vi "请双击登录.vi"() -> ()   [LabVIEW 2012]
panel:
  out "主VI路径":path
  out "注册状态提示":string
  in  "注册":bool
  in  "登录":bool
  in  "退出":bool
  in  "密    码":string
  in  "用户名":string
  out "数值":i32
  out "路径":path=path "D:/labVIs/0921/用户数据.txt"
  # "说明：请先输入用户名和密码再点击注册或登录\n默认用户名：20154207         密码：20154207"
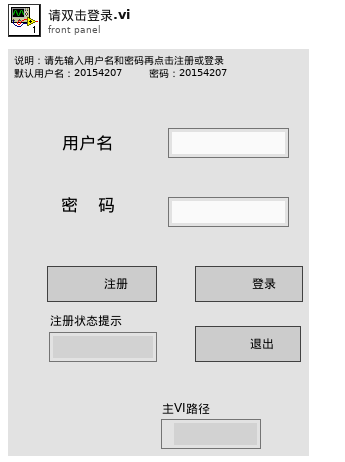
[diagram p1: front panel]
types:
  T1 = enum16{"open", "replace", "create", "open or create", "replace or create", "replace or create with confirmation"}
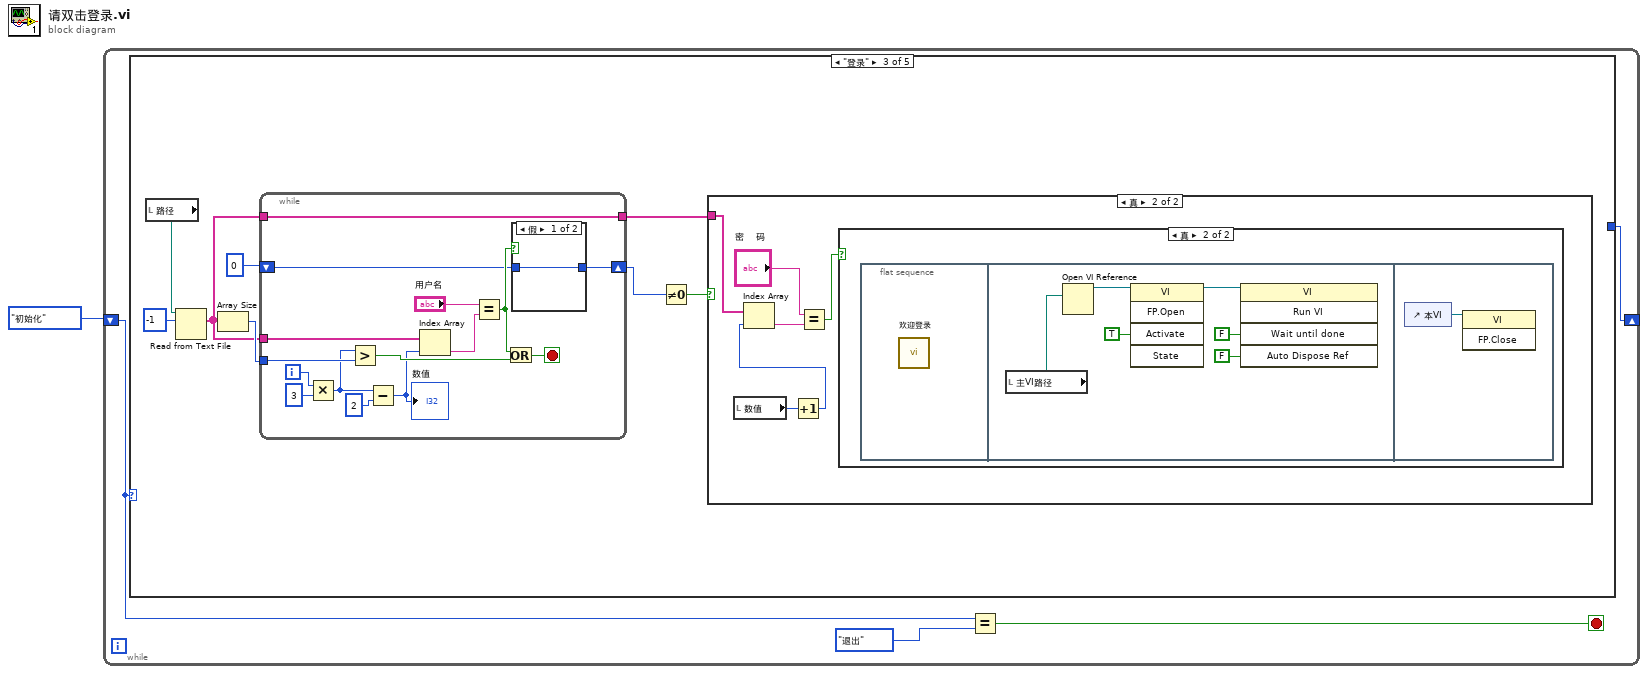
[diagram p0: block diagram]
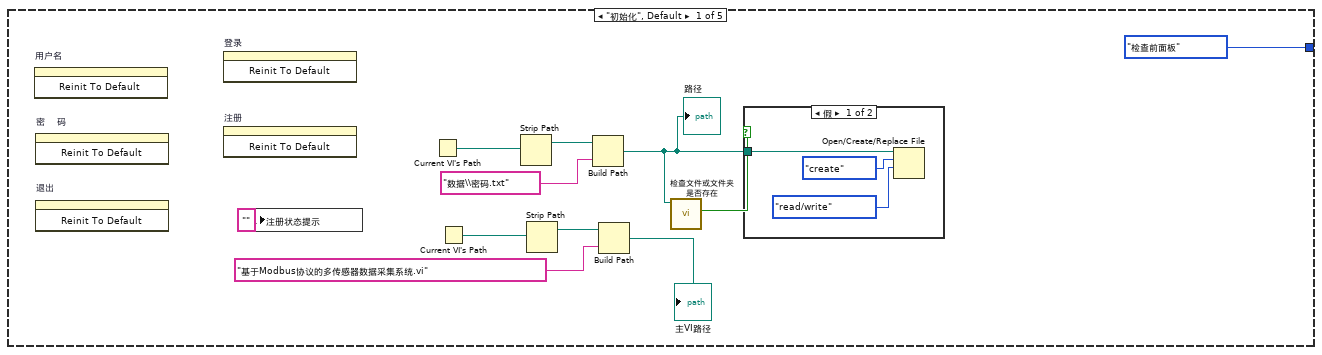
[diagram p2: hidden frame]
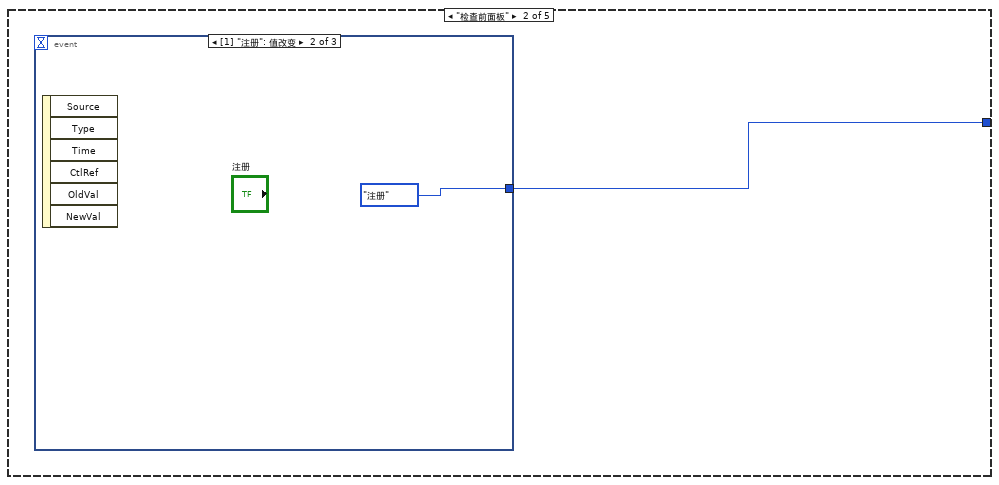
[diagram p4: hidden frame]
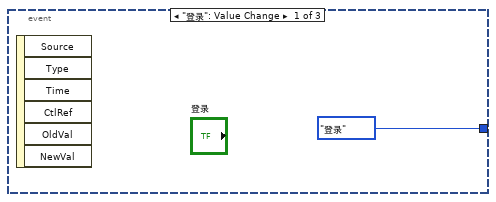
[diagram p5: hidden frame]
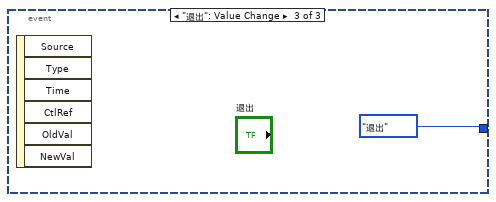
[diagram p6: hidden frame]
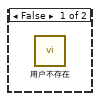
[diagram p7: hidden frame]
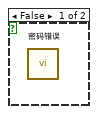
[diagram p8: hidden frame]
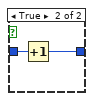
[diagram p9: hidden frame]
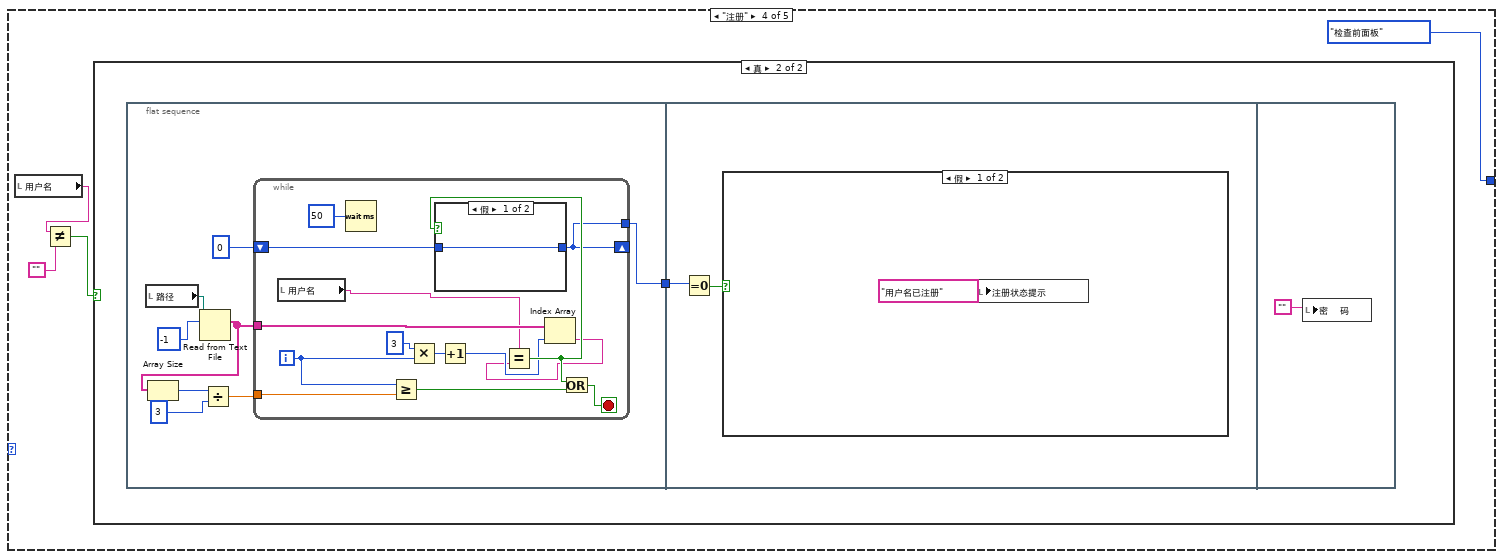
[diagram p10: hidden frame]
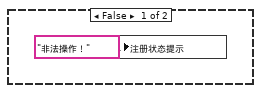
[diagram p11: hidden frame]
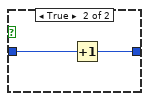
[diagram p12: hidden frame]
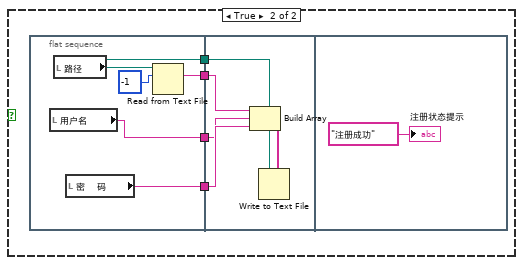
[diagram p13: hidden frame]
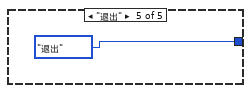
[diagram p14: hidden frame]
diagram:
  n1 = while {
    shift-right: [w5] -> _
    shift-left: enum16{"初始化", "检查前面板", "登录", "注册", "退出"}."初始化" ("枚举") -> [w3]
    stop <- w2 stop-if-true
    n2 = case shown="\"登录\"" w3 {
      tunnel: [enum16{"初始化", "检查前面板", "登录", "注册", "退出"}."检查前面板" ("枚举") w20 _ enum16{"初始化", "检查前面板", "登录", "注册", "退出"}."检查前面板" ("枚举") enum16{"初始化", "检查前面板", "登录", "注册", "退出"}."退出" ("枚举")] -> w5
      frame "初始化", Default {
        n3 = invoke on="用户名" class="Str" method="Reinit To Default"() -> ()  [unwired: 3 in, 3 out]
        n4 = invoke on="密    码" class="Str" method="Reinit To Default"() -> ()  [unwired: 3 in, 3 out]
        n5 = invoke on="退出" class="Bool" method="Reinit To Default"() -> ()  [unwired: 3 in, 3 out]
        n6 = invoke on="登录" class="Bool" method="Reinit To Default"() -> ()  [unwired: 3 in, 3 out]
        n7 = invoke on="注册" class="Bool" method="Reinit To Default"() -> ()  [unwired: 3 in, 3 out]
        n8 = local write "注册状态提示"("" ("注册状态")) -> ()
        n9 = Current VI's Path() -> (path=w15:path)
        n10 = Current VI's Path() -> (path=w9:path)
        n11 = Strip Path(path=w15) -> (stripped path=w14:path)  [unwired: 1 out]
        n12 = Strip Path(path=w9) -> (stripped path=w8:path)  [unwired: 1 out]
        n13 = Build Path(base path=w14, name or relative path="数据\\密码.txt" ("名称或相对路径")) -> (appended path=w12:path)
        "路径" <- w12
        n14 = Build Path(base path=w8, name or relative path="基于Modbus协议的多传感器数据采集系统.vi" ("名称或相对路径")) -> (appended path=→"主VI路径":path)
        n15 = call "检查文件或文件夹是否存在.vi"("path"=w12) -> ("file or folder exists?"=w16:bool)  [unwired: 8 in, 2 out]
        n16 = case shown="假" w16 {
          tunnel: w12 -> [w19 _]
          frame False {
            n17 = Open/Create/Replace File(file path (use dialog)=w19, operation (0:open)=T1."create" ("操作(0:open)"), access (0:read/write)=enum16{"read/write", "read-only", "write-only"}."read/write" ("权限(0:read/write)")) -> ()  [unwired: 3 in, 3 out]
          }
          frame True {
          }
        }
      }
      frame "检查前面板" {
        n18 = event shown="[1] \"注册\": 值改变" {
          selector: _ -> [_ _ _]
          dyn-events: _ -> [_ _ _]
          timeout: _ -> [_ _ _]
          tunnel: [enum16{"初始化", "检查前面板", "登录", "注册", "退出"}."登录" ("枚举") enum16{"初始化", "检查前面板", "登录", "注册", "退出"}."注册" ("枚举") enum16{"初始化", "检查前面板", "登录", "注册", "退出"}."退出" ("枚举")] -> w20
          event "登录": Value Change {
            n19 = event-data() -> ()  [unwired: 1 in, 6 out]
          }
          event "注册": Value Change {
            n20 = event-data() -> ()  [unwired: 1 in, 6 out]
          }
          event "退出": Value Change {
            n21 = event-data() -> ()  [unwired: 1 in, 6 out]
          }
        }
      }
      frame "登录" {
        n22 = local read "路径"() -> (w31:path)
        n23 = Read from Text File(file (use dialog)=w31, count=-1 ("计数")) -> (text=w25:string[])  [unwired: 2 in, 3 out]
        n24 = Array Size(array=w25) -> (size(s)=w26:i32)
        n25 = while {
          tunnel: w25 -> [w58]
          tunnel: w25 -> [w48]
          tunnel: w26 -> [w54]
          tunnel: [w48] -> w27
          shift-right: [w45] -> w29
          shift-left: 0 -> [w46]
          i -> [w52]
          stop <- w50 stop-if-true
          n26 = Multiply(x=w52, y=3) -> (x*y=w53:i32)
          n27 = Greater?(x=w53, y=w54) -> (0:w51:bool)
          n28 = Subtract(x=w53, y=2) -> (x-y=w49:i32)
          "数值" <- w49
          n29 = Index Array(array=w58, index=w49) -> (element=w57:string)
          n30 = Equal?(x="用户名", y=w57) -> (x = y?=w47:bool)
          n31 = Or(x=w47, y=w51) -> (x .or. y?=w50:bool)
          n32 = case shown="假" w47 {
            tunnel: w46 -> [w60 w62]
            tunnel: [w60 w61] -> w45
            frame False {
            }
            frame True {
              n33 = Increment(x=w62) -> (x+1=w61:i32)
            }
          }
        }
        n34 = Not Equal To 0?(x=w29) -> (x != 0?=w30:bool)
        n35 = case shown="真" w30 {
          tunnel: w27 -> [_ w35]
          frame False {
            n36 = call "用户不存在"() -> ()  [unwired: 10 in, 2 out]
          }
          frame True {
            n37 = local read "数值"() -> (w32:i32)
            n38 = Increment(x=w32) -> (x+1=w36:i32)
            n39 = Index Array(array=w35, index=w36) -> (element=w34:string)
            n40 = Equal?(x="密    码", y=w34) -> (x = y?=w33:bool)
            n41 = case shown="真" w33 {
              frame False {
                n42 = call "密码错误"() -> ()  [unwired: 10 in, 2 out]
              }
              frame True {
                n43 = flat-sequence {
                  frame #0 {
                    n44 = call "欢迎登录"() -> ()  [unwired: 10 in, 2 out]
                  }
                  frame #1 {
                    n45 = local read "主VI路径"() -> (w38:path)
                    n46 = Open VI Reference(vi path=w38) -> (vi reference=w39:refnum<vi>)  [unwired: 5 in, 1 out]
                    n47 = invoke class="VI" method="FP.Open"(reference=w39, "Activate"=TRUE) -> (reference out=w41:refnum<vi>)  [unwired: 3 in, 4 out]
                    n48 = invoke class="VI" method="Run VI"(reference=w41, "Wait until done"=FALSE, "Auto Dispose Ref"=FALSE) -> ()  [unwired: 2 in, 5 out]
                  }
                  frame #2 {
                    n49 = control-ref of="本VI"() -> (w44:refnum<vi>)
                    n50 = invoke class="VI" method="FP.Close"(reference=w44) -> ()  [unwired: 2 in, 3 out]
                  }
                }
              }
            }
          }
        }
      }
      frame "注册" {
        n51 = local read "用户名"() -> (w65:string)
        n52 = Not Equal?(x=w65, y="") -> (x != y?=w63:bool)
        n53 = case shown="真" w63 {
          frame False {
            n54 = local write "注册状态提示"("非法操作！" ("注册状态")) -> ()
          }
          frame True {
            n55 = flat-sequence {
              tunnel: [w70] -> w68
              tunnel: w68 -> [w95]
              frame #0 {
                n56 = local read "路径"() -> (w69:path)
                n57 = Read from Text File(file (use dialog)=w69, count=-1 ("计数")) -> (text=w73:string[])  [unwired: 2 in, 3 out]
                n58 = Array Size(array=w73) -> (size(s)=w75:i32)
                n59 = Divide(x=w75, y=3) -> (x/y=w71:dbl)
                n60 = while {
                  tunnel: w73 -> [w90]
                  shift-right: [w82] -> _
                  shift-left: 0 -> [w88]
                  tunnel: w71 -> [w86]
                  tunnel: [w82] -> w70
                  i -> [w80]
                  stop <- w83 stop-if-true
                  n61 = local read "用户名"() -> (w77:string)
                  n62 = Wait (ms)(milliseconds to wait=u32 50 ("等待时间（毫秒）")) -> ()  [unwired: 1 out]
                  n63 = Greater Or Equal?(x=w80, y=w86) -> (x >= y?=w84:bool)
                  n64 = Multiply(x=3, y=w80) -> (x*y=w87:i32)
                  n65 = Increment(x=w87) -> (x+1=w81:i32)
                  n66 = Index Array(array=w90, index=w81) -> (element=w79:string)
                  n67 = Equal?(x=w77, y=w79) -> (x = y?=w85:bool)
                  n68 = case shown="假" w85 {
                    tunnel: w88 -> [w91 w93]
                    tunnel: [w91 w92] -> w82
                    frame False {
                    }
                    frame True {
                      n69 = Increment(x=w93) -> (x+1=w92:i32)
                    }
                  }
                  n70 = Or(x=w85, y=w84) -> (x .or. y?=w83:bool)
                }
              }
              frame #1 {
                n71 = Equal To 0?(x=w95) -> (x = 0?=w94:bool)
                n72 = case shown="假" w94 {
                  frame False {
                    n73 = local write "注册状态提示"("用户名已注册") -> ()
                  }
                  frame True {
                    n74 = flat-sequence {
                      tunnel: [w102] -> w100
                      tunnel: [w101] -> w99
                      tunnel: [w104] -> w98
                      tunnel: [w103] -> w97
                      tunnel: w98 -> [w109]
                      tunnel: w99 -> [w106]
                      tunnel: w100 -> [w107]
                      tunnel: w97 -> [w108]
                      frame #0 {
                        n75 = local read "用户名"() -> (w101:string)
                        n76 = local read "路径"() -> (w103:path)
                        n77 = local read "密    码"() -> (w102:string)
                        n78 = Read from Text File(file (use dialog)=w103, count=-1 ("计数")) -> (text=w104:string)  [unwired: 2 in, 3 out]
                      }
                      frame #1 {
                        n79 = Build Array(w109, w106, w107) -> (w110:string[])
                        n80 = Write to Text File(file (use dialog)=w108, text=w110) -> ()  [unwired: 2 in, 3 out]
                      }
                      frame #2 {
                        "注册状态提示" <- "注册成功"
                      }
                    }
                  }
                }
              }
              frame #2 {
                n81 = local write "密    码"("") -> ()
              }
            }
          }
        }
      }
      frame "退出" {
      }
    }
    n82 = Equal?(x=w3, y=enum16{"初始化", "检查前面板", "登录", "注册", "退出"}."退出" ("枚举")) -> (x = y?=w2:bool)
  }
